vi "Launch.vi"(6 "AutoShutdown Slave (F)":bool, 7 "Clone if Reentrant (T)":bool=TRUE, 8 "error in":errorcluster, 11 "Parallel Process in":refnum<class "Parallel Process.lvclass">) -> (0 "error out":errorcluster, 1 "Already Running":bool, 3 "Parallel Process out":refnum<class "Parallel Process.lvclass">)   [LabVIEW 2011, in "Messenging.lvlib" / "Parallel Process.lvclass"]
doc: "Launches the \"Parallel Process\"."
uses:
  Parallel Process.lvclass
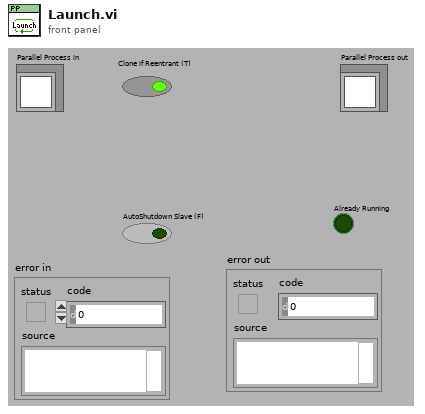
[diagram p1: front panel]
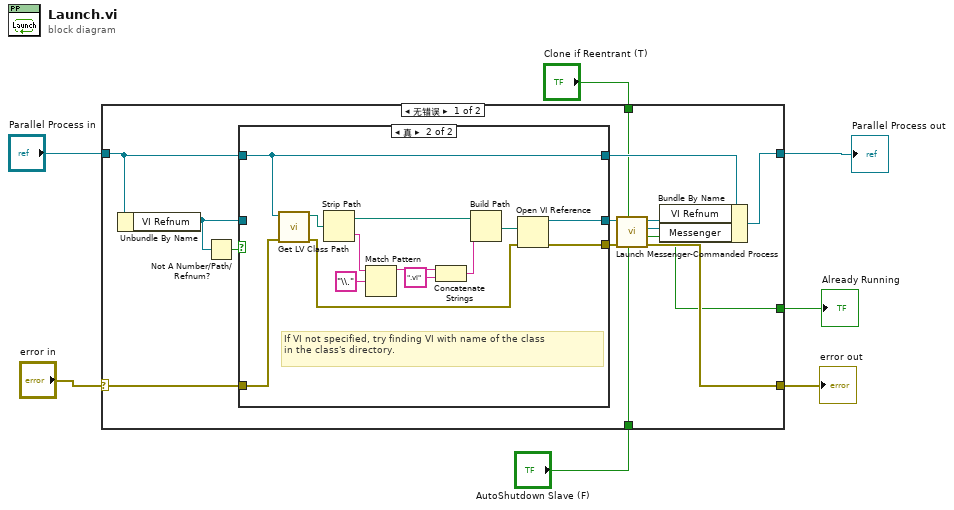
[diagram p0: block diagram]
diagram:
  n1 = case shown="无错误" "error in" {
    selector: "error in" -> [w15 w38]
    tunnel: [w21 w39] -> w7
    tunnel: [w18 w38] -> w6
    tunnel: "Parallel Process in" -> [w16 w39]
    tunnel: [w10 _] -> w3
    tunnel: "Clone if Reentrant (T)" -> [w9 _]
    tunnel: "AutoShutdown Slave (F)" -> [w8 _]
    frame No Error {
      n2 = Unbundle By Name(w16) -> ("VI Refnum"=w11:refnum<vi>)
      n3 = Not A Number/Path/Refnum?(number/path/refnum=w11) -> (NaN/Path/Refnum?=w17:bool)
      n4 = case shown="真" w17 {
        tunnel: w16 -> [w22 w26]
        tunnel: w15 -> [w23 w28]
        tunnel: [w23 w27] -> w14
        tunnel: [w22 w26] -> w13
        tunnel: [w24 w25] -> w12
        tunnel: w11 -> [w24 _]
        frame False {
        }
        frame True {
          # "If VI not specified, try finding VI with name of the class\nin the class's directory."
          n5 = call <vilib>:"Get LV Class Path.vi"("error in (no error)"=w28, "object"=w26) -> ("error out"=w29:errorcluster, "class path"=w37:path)  [unwired: 8 out]
          n6 = Strip Path(path=w37) -> (stripped path=w31:path, name=w36:string)
          n7 = Match Pattern(string=w36, regular expression="\\.") -> (before substring=w34:string)  [unwired: 4 out]
          n8 = Concatenate Strings(w34, ".vi" ("string")) -> (w32:string)
          n9 = Build Path(base path=w31, name or relative path=w32) -> (appended path=w30:path)
          n10 = Open VI Reference(vi path=w30, error in (no error)=w29) -> (vi reference=w25:refnum<vi>, error out=w27:errorcluster)  [unwired: 4 out]
        }
      }
      n11 = call "Launch Messenger-Commanded Process.vi"("Launch as Slave (F)"=w8, "Clone if Reentrant (T)"=w9, "error in"=w14, "VI Refnum"=w12) -> ("error out"=w18:errorcluster, "Already Running"=w10:bool, "Command Messenger"=w20:refnum<class "MGR.lvclass">, "vi reference"=w19:refnum<vi>)  [unwired: 4 out]
      n12 = Bundle By Name(cluster=w13, "VI Refnum"=w19, "Messenger"=w20) -> (w21:refnum<class "Parallel Process.lvclass">)
    }
    frame Error {
    }
  }
  "error out" <- w6
  "Parallel Process out" <- w7
  "Already Running" <- w3
